vi "LJLogM.vi"() -> ()   [LabVIEW 2022 SP3]
panel:
  out "ms per iteration":i32
  out "SerialNumber":i32
  out "ConnType":i32
  out "DevType":i32
  in  "Change Working Directory":bool
  in  "Max File Size (Bytes)":i32=1048576 min=1 max=2000000000
  in  "Graph?":bool[](array[boolean])
  out "Waveform Graph":cluster{dbl, dbl, dbl[][]}(graph)
  in  "Graph History":i32=1000 min=0
  in  "exit":bool
  out "Scaled":dbl[](array[numeric]) format="%.6f"
  in  "Scaling Equation":string[](array[string])=["y=v0", "y=v1", "y=v2", "y=v3", "y=v4", "y=v5", "y=v6", "y=v7"]
  in  "# Channels":i32=4 min=1 max=16
  out "Value":dbl[](array[numeric]) format="%.6f"
  in  "Name":string[](array[string])=["0", "1", "2", "3", "4", "5", "6", "7"]
  out "# of iterations":i32
  in  "Interval (ms)":u32=500
  out "Current Data File":path
  in  "Data File Prefix":string="data"
  in  "Write To File":bool
  out "Error Message":string
  # "0"
  # "1"
  # "2"
  # "3"
  # "To configure inputs,\nexit this program and\nuse the \"IO Config\" tab\nin Kipling.  To control\nopening, edit the file\nljlogm_open.cfg."
  # "4"
  # "5"
  # "6"
  # "7"
  # "8"
  # "9"
  # "10"
  # "11"
  # "12"
  # "13"
  # "14"
  # "15"
  # "-\"a\" - \"p\" correspond to the raw Voltage value\n  from the 1st through 16th row.\n-The scaled output value is \"y\".\n-If your equation has an error, the output\n  will be zero."
  # "# scans"
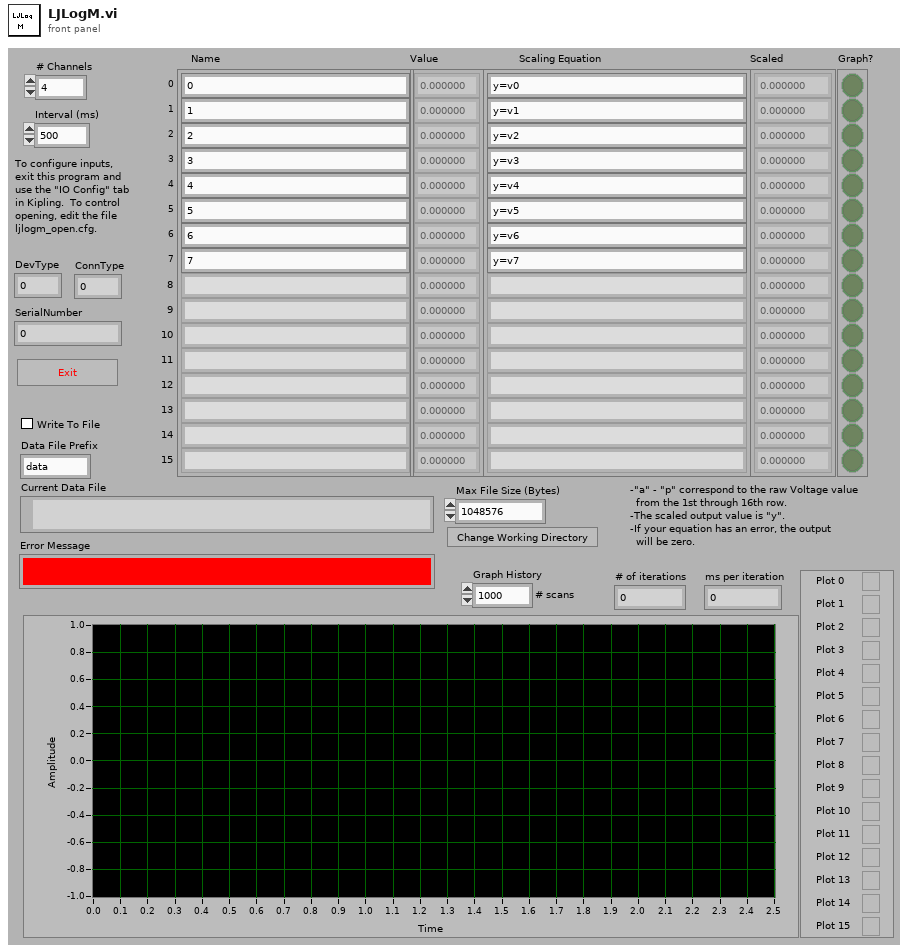
[diagram p1: front panel]
types:
  T1 = cluster{"+Ch":string[], "-Ch":string[], "Ranges":u16[], "Scaling Equation":string[], "Graph?":bool[]}
  T2 = cluster{"# Channels":i32, "Name":string[], string[], u16[], "Scaling Equation":string[]}
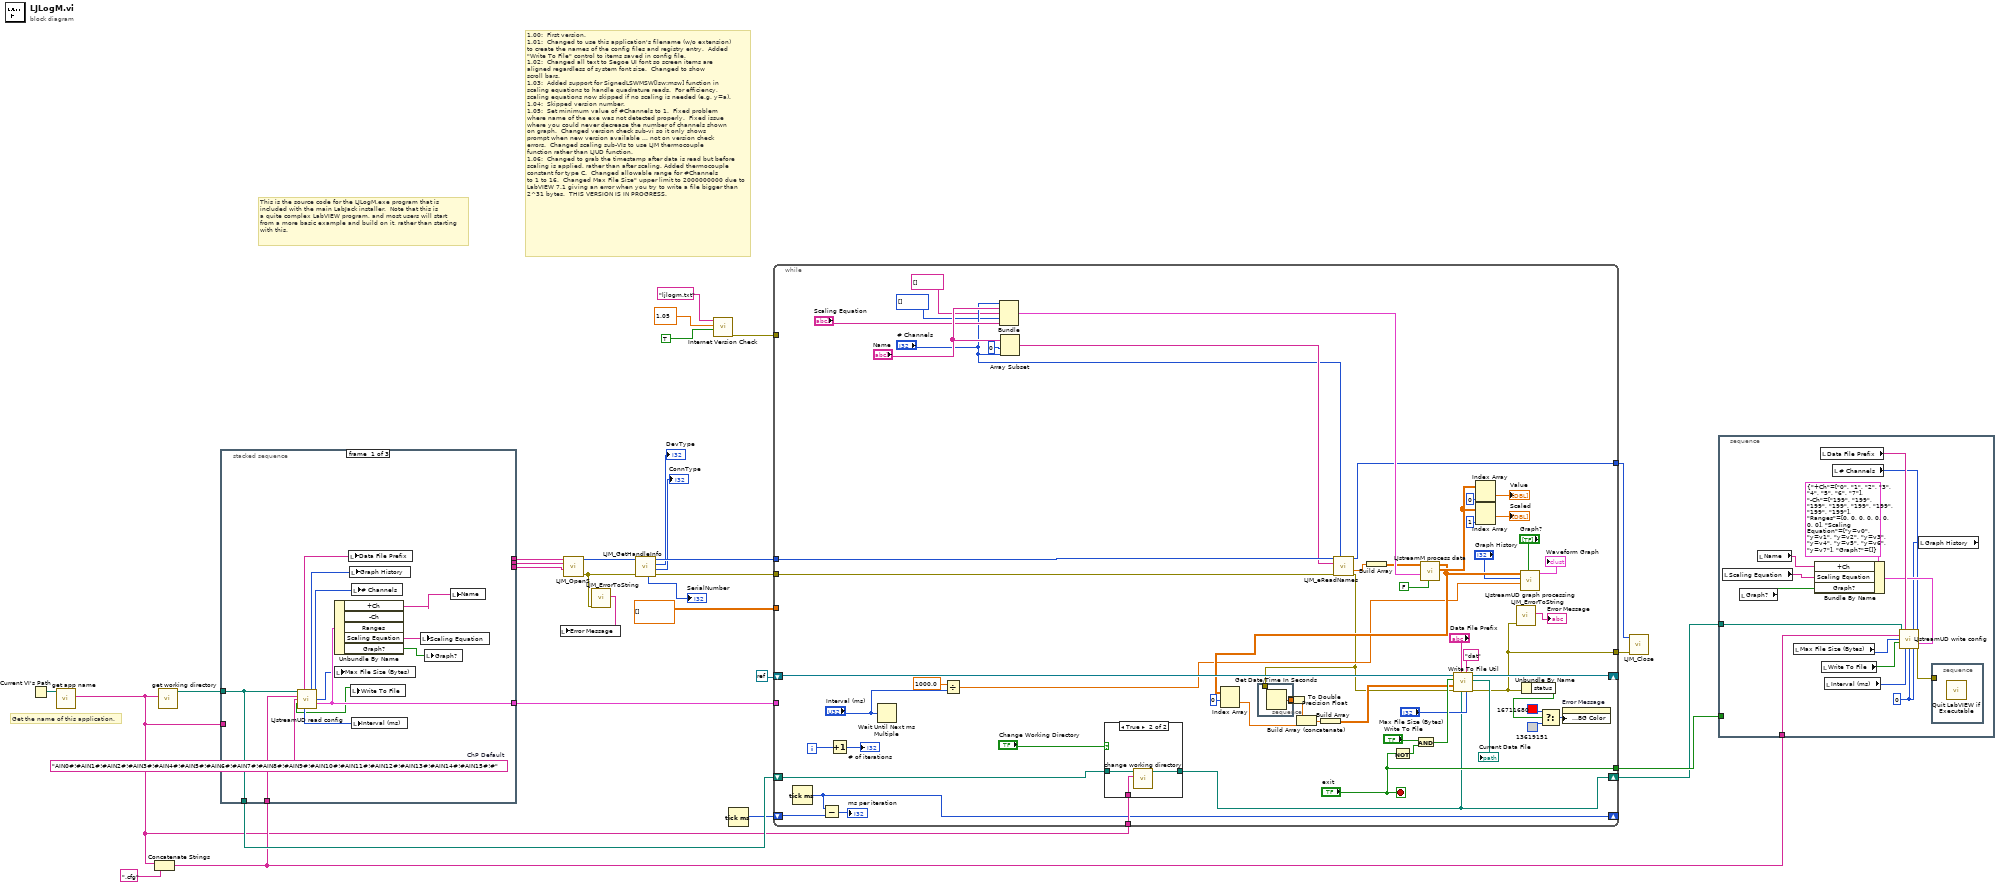
[diagram p0: block diagram]
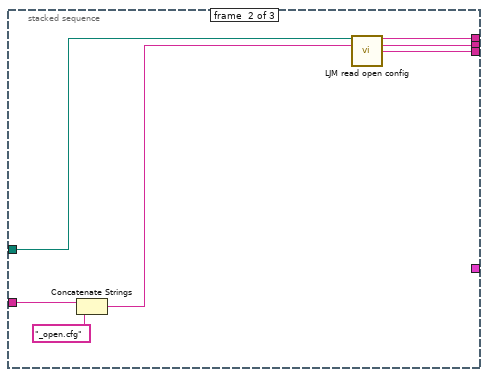
[diagram p3: hidden frame]
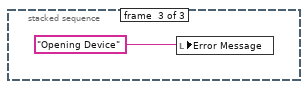
[diagram p4: hidden frame]
diagram:
  # "This is the source code for the LJLogM.exe program that is\nincluded with the main LabJack installer.  Note that this is \na quite complex LabVIEW program, and most users will start\nfrom a more basic example and build on it, rather than starting\nwith this."
  # "Get the name of this application."
  # "1.00:  First version.\n1.01:  Changed to use this application's filename (w/o extension)\nto create the names of the config files and registry entry.  Added\n\"Write To File\" control to items saved in config file.\n1.02:  Changed all text to Segoe UI font so screen items are\naligned regardless of system font size.  Changed to show\nscroll bars.\n1.03:  Added support for SignedLSWMSW[lsw:msw] function in\nscaling equations to handle quadrature reads.  For efficiency,\nscaling equations now skipped if no scaling is needed (e.g. y=a).\n1.04:  Skipped version number.\n1.05:  Set minimum value of #Channels to 1.  Fixed problem\nwhere name of the exe was not detected properly.  Fixed issue\nwhere you could never decrease the number of channels shown\non graph.  Changed version check sub-vi so it only shows\nprompt when new version available ... not on version check\nerrors.  Changed scaling sub-VIs to use LJM thermocouple\nfunction rather than LJUD function.\n1.06:  Changed to grab the timestamp after data is read but before\nscaling is applied, rather than after scaling. Added thermocouple\nconstant for type C.  Changed allowable range for #Channels\nto 1 to 16.  Changed Max File Size\" upper limit to 2000000000 due to\nLabVIEW 7.1 giving an error when you try to write a file bigger than\n2^31 bytes.  THIS VERSION IS IN PROGRESS."
  n1 = Current VI's Path() -> (path=w5:path)
  n2 = call "get app name.vi"("Current VI's Path"=w5) -> ("App Name Without Extension"=w4:string)  [unwired: 4 in, 2 out]
  n3 = Concatenate Strings(w4, ".cfg" ("filename")) -> (w7:string)
  n4 = call "get working directory.vi"("Application Name"=w4) -> ("Working Directory"=w16:path)  [unwired: 9 in, 1 out]
  n5 = stacked-sequence {
    tunnel: [w42 _ _] -> w27
    tunnel: [w33 _ _] -> w24
    tunnel: w16 -> [w33 w46 _]
    tunnel: [_ w49 _] -> w15
    tunnel: [_ w48 _] -> w14
    tunnel: [_ w47 _] -> w13
    tunnel: w7 -> [w31 _ _]
    tunnel: w4 -> [_ w44 _]
    frame #0 {
      w32 = "AIN0#!#AIN1#!#AIN2#!#AIN3#!#AIN4#!#AIN5#!#AIN6#!#AIN7#!#AIN8#!#AIN9#!#AIN10#!#AIN11#!#AIN12#!#AIN13#!#AIN14#!#AIN15#!#"  # ChP Default
      n6 = call "LJstreamUD read config.vi"("Working Directory"=w33, "filename"=w31, "ChP Default"=w32) -> ("Data File Prefix"=w39:string, "Graph History"=w35:i32, "# Channels"=w37:i32, "Max File Size (Bytes)"=w34:i32, "Write To File"=w30:bool, "Channel Setup"=w42:T1, "Interval (ms)"=w38:u32)  [unwired: 1 in, 5 out]
      n7 = Unbundle By Name(w42) -> ("+Ch"=w40:string[], "Scaling Equation"=w41:string[], "Graph?"=w36:bool[])  [unwired: 2 out]
      n8 = local write "Max File Size (Bytes)"(w34) -> ()
      n9 = local write "Data File Prefix"(w39) -> ()
      n10 = local write "Graph History"(w35) -> ()
      n11 = local write "Write To File"(w30) -> ()
      n12 = local write "# Channels"(w37) -> ()
      n13 = local write "Interval (ms)"(w38) -> ()
      n14 = local write "Scaling Equation"(w41) -> ()
      n15 = local write "Graph?"(w36) -> ()
      n16 = local write "Name"(w40) -> ()
    }
    frame #1 {
      n17 = Concatenate Strings(w44, "_open.cfg" ("filename")) -> (w43:string)
      n18 = call "LJM read open config.vi"("Working Directory"=w46, "filename"=w43) -> ("DeviceType"=w49:string, "ConnectionType"=w48:string, "Identifier"=w47:string)  [unwired: 10 in, 1 out]
    }
    frame #2 {
      n19 = local write "Error Message"("Opening Device" ("Error Message")) -> ()
    }
  }
  n20 = call "LJM_OpenS.vi"("Identifier"=w13, "ConnectionType"=w14, "DeviceType"=w15) -> ("error out"=w12:errorcluster, "Handle"=w20:i32)  [unwired: 7 in]
  n21 = call "LJM_ErrorToString.vi"("error in"=w12) -> ("String"=w11:string)  [unwired: 10 in]
  n22 = local write "Error Message"(w11) -> ()
  n23 = call "LJM_GetHandleInfo.vi"("error in"=w12, "Handle In"=w20) -> ("error out"=w22:errorcluster, "ConnectionType"=→"ConnType":i32, "DeviceType"=→"DevType":i32, "Handle Out"=w21:i32, "SerialNumber"=→"SerialNumber":i32)  [unwired: 2 in, 3 out]
  n24 = call "Internet Version Check.vi"("Prompt If Newer Version Available"=TRUE, "Version In"=1.05, "Version File Name"="ljlogm.txt") -> ("error out"=w26:errorcluster)  [unwired: 6 in, 2 out]
  n25 = Tick Count (ms)() -> (millisecond timer value=w6:u32)
  n26 = while {
    shift-left: w24 -> [w65]
    shift-right: [w64] -> w23
    tunnel: w4 -> [w66]
    tunnel: w26 -> [_]
    tunnel: dbl[][] [] ("Waveform Chart") -> [_]
    tunnel: w22 -> [w62]
    tunnel: w21 -> [w63]
    shift-left: refnum<k0> refnum -> [w94]
    shift-right: [w96] -> _
    tunnel: w27 -> [_]
    tunnel: ["exit"] -> w25
    tunnel: [w56] -> w10
    tunnel: [w55] -> w9
    shift-right: [w52] -> _
    shift-left: w6 -> [w54]
    i -> [w101]
    stop <- "exit" stop-if-true
    n27 = Tick Count (ms)() -> (millisecond timer value=w52:u32)
    n28 = Subtract(x=w52, y=w54) -> (x-y=→"ms per iteration":u32)
    n29 = Increment(x=w101) -> (x+1=→"# of iterations":i32)
    n30 = Wait Until Next ms Multiple(millisecond multiple="Interval (ms)") -> ()  [unwired: 1 out]
    n31 = Divide(x=1000.0, y="Interval (ms)") -> (x/y=w74:dbl)
    n32 = Bundle("# Channels"="# Channels", "Name"="Name", string[] [], u16[] [], "Scaling Equation"="Scaling Equation") -> (w91:T2)  [unwired: 1 in]
    n33 = Array Subset(array="Name", index=0 ("Array Index"), length="# Channels") -> (w61:string[])
    n34 = case shown="True" "Change Working Directory" {
      tunnel: w66 -> [_ w111]
      tunnel: w65 -> [w108 w110]
      tunnel: [w108 w109] -> w64
      frame False {
      }
      frame True {
        n35 = call "change working directory.vi"("Application Name"=w111, "Working Directory In"=w110) -> ("Working Directory Out"=w109:path)  [unwired: 9 in]
      }
    }
    n36 = call "LJM_eReadNames.vi"("Handle In"=w63, "NumFrames (Auto-Detect)"="# Channels", "aNames"=w61, "error in"=w62) -> ("Handle Out"=w55:i32, "aValuesOut"=w57:dbl[], "error out"=w51:errorcluster)  [unwired: 8 in, 1 out]
    n37 = stacked-sequence {
      tunnel: [w113] -> w88
      tunnel: w51 -> [_]
      frame #0 {
        n38 = Get Date/Time In Seconds() -> (seconds since 1Jan1904=w112:timestamp)
        n39 = To Double Precision Float(number=w112) -> (double precision float=w113:dbl)
      }
    }
    n40 = Build Array(w57) -> (w86:dbl[][])
    n41 = Not(x="exit") -> (.not. x?=w103:bool)
    n42 = And(x="Write To File", y=w103) -> (x .and. y?=w95:bool)
    n43 = call "LJstreamM process data.vi"("Disable Scaling"=FALSE, "Channel Config"=w91, "Voltages"=w86) -> ("Volts,Scaled Averages"=w90:dbl[][], "Scaled Data"=w79:dbl[][])  [unwired: 7 in]
    n44 = Index Array(array=w79, index (row)=0 ("Index (row)")) -> (element=w84:dbl[])  [unwired: 1 in]
    n45 = Build Array (concatenate)(w88, w84) -> (w87:dbl[])
    n46 = Build Array(w87) -> (w83:dbl[][])
    n47 = call "Write To File Util.vi"("Maximum File Size (Bytes)"="Max File Size (Bytes)", "Data File Extension"="dat", "Working Directory"=w64, "Data File Prefix"="Data File Prefix", "error in"=w51, "Data"=w83, "Write To File"=w95, "File Refnum In"=w94) -> ("error out"=w56:errorcluster, "Current Data File"=→"Current Data File":path, "File Refnum Out"=w96:refnum<file>)  [unwired: 1 in]
    n48 = Index Array(array=w90, index (col)=0 ("Disabled Index (col)")) -> (element=→"Value":dbl[])  [unwired: 1 in]
    n49 = Index Array(array=w90, index (col)=1 ("Disabled Index (col)")) -> (element=→"Scaled":dbl[])  [unwired: 1 in]
    n50 = call "LJM_ErrorToString.vi"("error in"=w56) -> ("String"=→"Error Message":string)  [unwired: 10 in]
    n51 = call "LJstreamUD graph processing.vi"("Graph?"="Graph?", "Scan Rate"=w74, "Graph History (# scans)"="Graph History", "Scaled Data"=w79) -> ("Graph Data"=→"Waveform Graph":cluster{dbl, dbl, dbl[][]})  [unwired: 7 in]
    n52 = Unbundle By Name(w56) -> ("status"=w71:bool)
    n53 = Select(t=u32 16711680, s=w71, f=u32 13619151) -> (s? t:f=w70:u32)
    n54 = property on="Error Message" class="Str"("Text.Text Colors:BG Color"=w70) -> ()  [unwired: 2 in, 2 out]
  }
  n55 = call "LJM_Close.vi"("error in"=w10, "Handle"=w9) -> ()  [unwired: 9 in, 1 out]
  n56 = stacked-sequence {
    tunnel: w23 -> [w119]
    tunnel: w25 -> [_]
    tunnel: w7 -> [w115]
    frame #0 {
      w116 = u8 0 ("Resolution")
      n57 = local read "Scaling Equation"() -> (w123:string[])
      n58 = local read "Graph?"() -> (w122:bool[])
      n59 = local read "Name"() -> (w124:string[])
      n60 = local read "Max File Size (Bytes)"() -> (w118:i32)
      n61 = Bundle By Name(cluster=T1 {"+Ch"=["0", "1", "2", "3", "4", "5", "6", "7"], "-Ch"=["199", "199", "199", "199", "199", "199", "199", "199"], "Ranges"=[0, 0, 0, 0, 0, 0, 0, 0], "Scaling Equation"=["y=v0", "y=v1", "y=v2", "y=v3", "y=v4", "y=v5", "y=v6", "y=v7"], "Graph?"=[]} ("Channel Setup"), "+Ch"=w124, "Scaling Equation"=w123, "Graph?"=w122) -> (w121:T1)
      n62 = local read "Data File Prefix"() -> (w127:string)
      n63 = local read "Write To File"() -> (w114:bool)
      n64 = local read "Interval (ms)"() -> (w126:u32)
      n65 = local read "# Channels"() -> (w120:i32)
      n66 = local read "Graph History"() -> (w117:i32)
      n67 = call "LJstreamUD write config.vi"("Working Directory"=w119, "Data File Prefix"=w127, "Graph History"=w117, "# Channels"=w120, "filename"=w115, "Max File Size (Bytes)"=w118, "Write To File"=w114, "Channel Setup"=w121, "Interval (ms)"=w126, "Resolution"=w116, "SettlingFactor"=w116) -> ("error out"=w128:errorcluster)  [unwired: 4 in]
      n68 = stacked-sequence {
        tunnel: w128 -> [_]
        frame #0 {
          n69 = call "Quit LabVIEW if Executable.vi"() -> ()  [unwired: 1 in]
        }
      }
    }
  }
